vi "Process.vi"(8 "error in":errorcluster, 11 "Example Instrument UI":refnum<class "Instrument UI.Framework-Template.lvclass">) -> (0 "error out":errorcluster, 3 "Example Instrument UI out":refnum<class "Instrument UI.Framework-Template.lvclass">)   [LabVIEW 2019, in "Instrument UI.Framework-Template.lvclass"]
doc: "---------------------------------------------------------------\nJKI State Machine Objects™\nhttp://jki.net/state-machine-objects/\nCopyright (C) 2005-2015, JKI <info@jki.net>\nALL RIGHTS RESERVEDJKI State Machine Objects (SMO) 1.0.0.5\nJKI - JKI\nCopyright (c) 2016, JKI"
uses:
  Instrument UI.Framework-Template.lvclass
  C:/Program Files (x86)/National Instruments/LabVIEW 2019/vi.lib/JKI/JKI SMO/SMO/SMO.lvclass
  C:/Program Files (x86)/National Instruments/LabVIEW 2019/user.lib/LevyLab/Instrument Framework/SMOs/Instrument UI/Instrument UI.lvclass
  C:/Program Files (x86)/National Instruments/LabVIEW 2019/vi.lib/JKI/JKI SMO/SMO.UI/SMO.UI.lvclass
  Instrument.Framework-Template/Typedefs/Instrument.Framework-Template.getAll--Cluster.ctl
  Instrument.Framework-Template/Instrument.Framework-Template.lvclass
  C:/Program Files (x86)/National Instruments/LabVIEW 2019/user.lib/LevyLab/Instrument Framework/SMOs/Instrument/Instrument.lvclass
  Instrument UI.Framework-Template.UI--Cluster.ctl
  Instrument.Framework-Template/Typedefs/Instrument.Framework-Template.Configuration--Cluster.ctl
  <userlib>/LevyLab/Instrument Framework/SMOs/Configuration/Configuration.lvclass
  <userlib>/LevyLab/Instrument Framework/SMOs/Instrument UI/Instrument UI.lvclass/Instrument UI.ctl
  <vilib>/JKI/JKI SMO/SMO/SMO.lvclass/SMO.ctl
  <userlib>/LevyLab/Instrument Framework/SMOs/Configuration/Configuration.lvclass/Configuration.ctl
  <userlib>/LevyLab/Instrument Framework/SMOs/Instrument/Instrument.lvclass/Instrument.ctl
  <userlib>/LevyLab/Instrument Framework/SMOs/Instrument/Typedefs/Client Type--Enum.ctl
  614f1787-3484-4d72-b522-1f8c221dac07.vi
  064e3a37-d4cf-416d-9c97-81a00de9d50c.vi
  <vilib>/JKI/JKI SMO/SMO/Private/ReftoDVR--SMO.vi
  614f1787-3484-4d72-b522-1f8c221dac07.vi/6126265b-52a9-4036-b9ab-d7def26448fd.vi
  064e3a37-d4cf-416d-9c97-81a00de9d50c.vi/2934c5b6-9d9a-4612-aef0-474eff5135e3.vi
  614f1787-3484-4d72-b522-1f8c221dac07.vi/6126265b-52a9-4036-b9ab-d7def26448fd.vi/3777206e-62d3-4194-bbb6-d708f28c6636.vi
  <userlib>/LevyLab/Instrument Framework/SMOs/Instrument/API/Send and Receive.vi
  614f1787-3484-4d72-b522-1f8c221dac07.vi/6126265b-52a9-4036-b9ab-d7def26448fd.vi/c2acc09a-a3b2-411f-96f0-93bdcc04d904.vi
  <userlib>/LevyLab/Instrument Framework/SMOs/Instrument/Private/Get Client Type.vi
  064e3a37-d4cf-416d-9c97-81a00de9d50c.vi/2934c5b6-9d9a-4612-aef0-474eff5135e3.vi/d31bd197-f2cf-45ec-b348-66ecc1fb7fa3.vi
  064e3a37-d4cf-416d-9c97-81a00de9d50c.vi/2934c5b6-9d9a-4612-aef0-474eff5135e3.vi/bcf0d896-5092-4459-a902-822cb84f3d2f.vi
  614f1787-3484-4d72-b522-1f8c221dac07.vi/6126265b-52a9-4036-b9ab-d7def26448fd.vi/3777206e-62d3-4194-bbb6-d708f28c6636.vi/a171245e-ace2-4a31-ad0e-c1ba96aac09f.vi
  614f1787-3484-4d72-b522-1f8c221dac07.vi/6126265b-52a9-4036-b9ab-d7def26448fd.vi/3777206e-62d3-4194-bbb6-d708f28c6636.vi/314606e5-fab2-4c4b-855f-38e561406072.vi
  614f1787-3484-4d72-b522-1f8c221dac07.vi/6126265b-52a9-4036-b9ab-d7def26448fd.vi/c2acc09a-a3b2-411f-96f0-93bdcc04d904.vi/068c89fb-261c-4114-b3e0-8879b2039521.vi
  614f1787-3484-4d72-b522-1f8c221dac07.vi/6126265b-52a9-4036-b9ab-d7def26448fd.vi/c2acc09a-a3b2-411f-96f0-93bdcc04d904.vi/70e8e4d8-081c-4447-abab-7ffc08a24431.vi
  064e3a37-d4cf-416d-9c97-81a00de9d50c.vi/2934c5b6-9d9a-4612-aef0-474eff5135e3.vi/d31bd197-f2cf-45ec-b348-66ecc1fb7fa3.vi/16df6886-ccac-4f12-823d-852507d7b6d3.vi
  064e3a37-d4cf-416d-9c97-81a00de9d50c.vi/2934c5b6-9d9a-4612-aef0-474eff5135e3.vi/d31bd197-f2cf-45ec-b348-66ecc1fb7fa3.vi/d363edf0-f48d-4095-b52d-a98fc5c23e31.vi
  064e3a37-d4cf-416d-9c97-81a00de9d50c.vi/2934c5b6-9d9a-4612-aef0-474eff5135e3.vi/bcf0d896-5092-4459-a902-822cb84f3d2f.vi/3efd9854-12da-426d-b303-5f5dfdd99cd3.vi
  064e3a37-d4cf-416d-9c97-81a00de9d50c.vi/2934c5b6-9d9a-4612-aef0-474eff5135e3.vi/bcf0d896-5092-4459-a902-822cb84f3d2f.vi/021688bb-175a-4f04-92c2-7b75fc3f16e3.vi
  614f1787-3484-4d72-b522-1f8c221dac07.vi/6126265b-52a9-4036-b9ab-d7def26448fd.vi/c2acc09a-a3b2-411f-96f0-93bdcc04d904.vi/068c89fb-261c-4114-b3e0-8879b2039521.vi/f4340ad4-3f7d-43fc-a5b8-8cfecf0320e0.vi
  614f1787-3484-4d72-b522-1f8c221dac07.vi/6126265b-52a9-4036-b9ab-d7def26448fd.vi/c2acc09a-a3b2-411f-96f0-93bdcc04d904.vi/068c89fb-261c-4114-b3e0-8879b2039521.vi/09137493-ac28-451c-9813-f227a1b20a03.vi
  064e3a37-d4cf-416d-9c97-81a00de9d50c.vi/2934c5b6-9d9a-4612-aef0-474eff5135e3.vi/bcf0d896-5092-4459-a902-822cb84f3d2f.vi/3efd9854-12da-426d-b303-5f5dfdd99cd3.vi/ec8d0cc2-9f9f-4698-9277-550a01addf9f.vi
  064e3a37-d4cf-416d-9c97-81a00de9d50c.vi/2934c5b6-9d9a-4612-aef0-474eff5135e3.vi/bcf0d896-5092-4459-a902-822cb84f3d2f.vi/3efd9854-12da-426d-b303-5f5dfdd99cd3.vi/599ad89e-f603-4806-a637-659fe558540e.vi
  <userlib>/LevyLab/Instrument Framework/SMOs/Instrument/Private/Get RC Connection Status.vi
  <userlib>/LevyLab/Instrument Framework/SMOs/Instrument/API/Enum to String.vi
  <userlib>/LevyLab/Instrument Framework/SMOs/RemoteControl/API/Send and Receive.vi
  <vilib>/Utility/Data Type/Get Type Information.vi
  <vilib>/JDP Science/JSONtext/JSON text to Variant.vi
  <vilib>/JDP Science/JSONtext/Variant to JSON Text.vi
  <vilib>/National Instruments/GUID Generator/Guid Generator.vi
  <userlib>/LevyLab/Instrument Framework/SMOs/Instrument/Private/Instrument.MessageFromProcess.EventStructure.vi
  <userlib>/LevyLab/Instrument Framework/SMOs/Instrument/Instrument.lvclass
  <vilib>/JDP Science/JSONtext/LVClass Serializer/JSONtext LVClass Serializer.lvclass
  <userlib>/LevyLab/Instrument Framework/SMOs/Instrument UI/Instrument UI.lvclass
  <vilib>/JKI/JKI SMO/SMO/SMO.lvclass
  <vilib>/JKI/JKI SMO/SMO.UI/SMO.UI.lvclass
panel:
  in  "Parameter 2":string
  out "Numeric":u32
  in  "Set Parameter":bool
  in  "Parameter":dbl
  in  "STOP":bool
  out "SMO string":string
  out "SMO Boolean":bool
  out "Logger SMO":dbl
  out "Levy 1":dbl
  # "#todo\nmake UI here. maybe include a nice picture of the hardware?"
  # "#todo\nadd buttons to do stuff (e.g., change a setting)\nButtons should trigger an event"
  # "#todo\nresize this box if you want your UI to be different size"
  # "SMO UI Template"
  # "For instructions on how to use the JKI State Machine Objects, examples and video tutorials, visit:\nhttp://jki.net/state-machine-objects/\n\nJKI State Machine Objects™\nhttp://jki.net/state-machine-objects/\nCopyright (C) 2005-2015, JKI <info@jki.net>\nALL RIGHTS RESERVED"
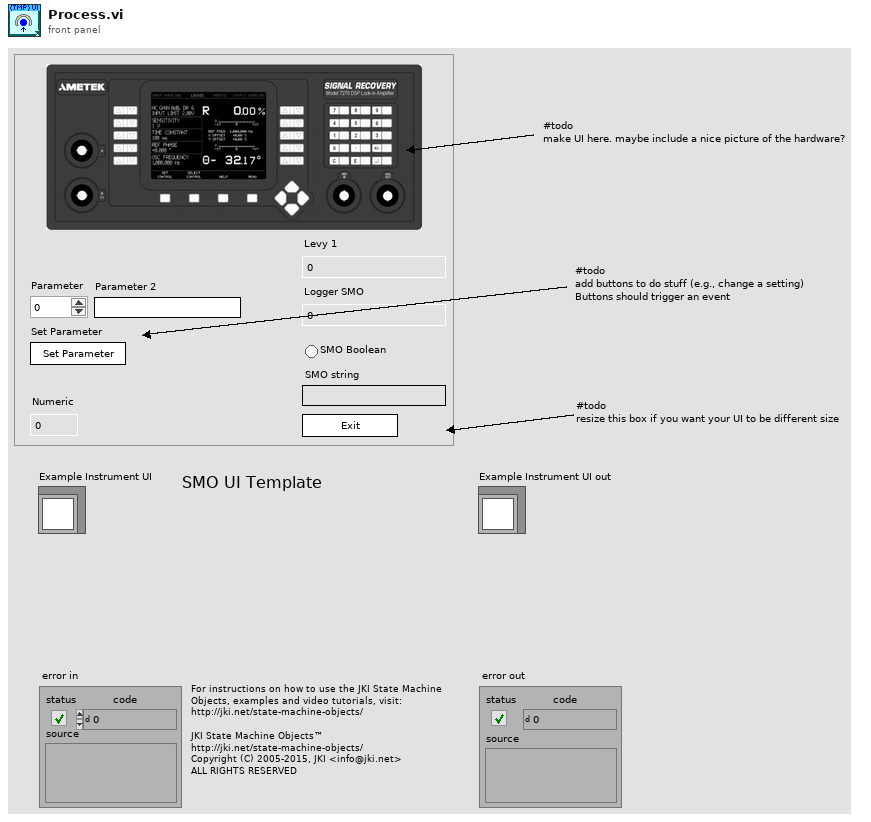
[diagram p1: front panel]
types:
  T1 = enum32{"invalid app kind", "Development System", "Run Time System", "Student Edition", "Embedded LabVIEW", "Evaluation", "Custom"}
  T2 = enum32{"Invalid", "Standard", "Closed", "Hidden", "Minimized", "Maximized"}
  T3 = typedef "Instrument.lvclass/Client Type--Enum.ctl" = enum16{"Remote", "Local"}
  T4 = typedef "Instrument.Framework-Template.lvclass/Instrument.Framework-Template.Configuration--Cluster.ctl" = cluster{"Example Setting 1":dbl, "Example Setting 2":dbl, "Example Setting 3":string}
  T5 = typedef "Instrument.Framework-Template.lvclass/Instrument.Framework-Template.getAll--Cluster.ctl" = cluster{"Levy 1":dbl, "Logger SMO":dbl, "SMO Boolean":bool, "SMO String":string}
  T6 = typedef "Instrument UI.Framework-Template.lvclass/Instrument UI.Framework-Template.UI--Cluster.ctl" = cluster{"Parameter":dbl, "Parameter 2":string}
  T7 = cluster{"Core":cluster{"Current VI Reference":refnum<vi>, "Close Panel on Exit?":bool, "Last Error":cluster{"error":errorcluster, "previous state":string, "remaining states":string}, "Shutdown?":bool}, "Instrument UI":refnum<class "Instrument UI.Framework-Template.lvclass">, "Instrument":refnum<class "Instrument.Framework-Template.lvclass">, "Configuration":refnum<class "Configuration.lvclass">, "Config Cluster":T4, "getAll":T5, "UI Cluster":T6}
  T8 = cluster{"Current VI Reference":refnum<vi>, "Close Panel on Exit?":bool, "Last Error":cluster{"error":errorcluster, "previous state":string, "remaining states":string}, "Shutdown?":bool}
  T9 = typedef "SMO.lvclass/Protected Events.ctl" = cluster{"StopProcesses":refnum<user-event>, "AbortProcesses":refnum<user-event>, "Config Changed":refnum<user-event>, "Dependency":refnum<user-event>}
  T10 = typedef "Instrument.lvclass/PublicEvents--Cluster.ctl" = cluster{"MessageFromProcess":refnum<user-event>}
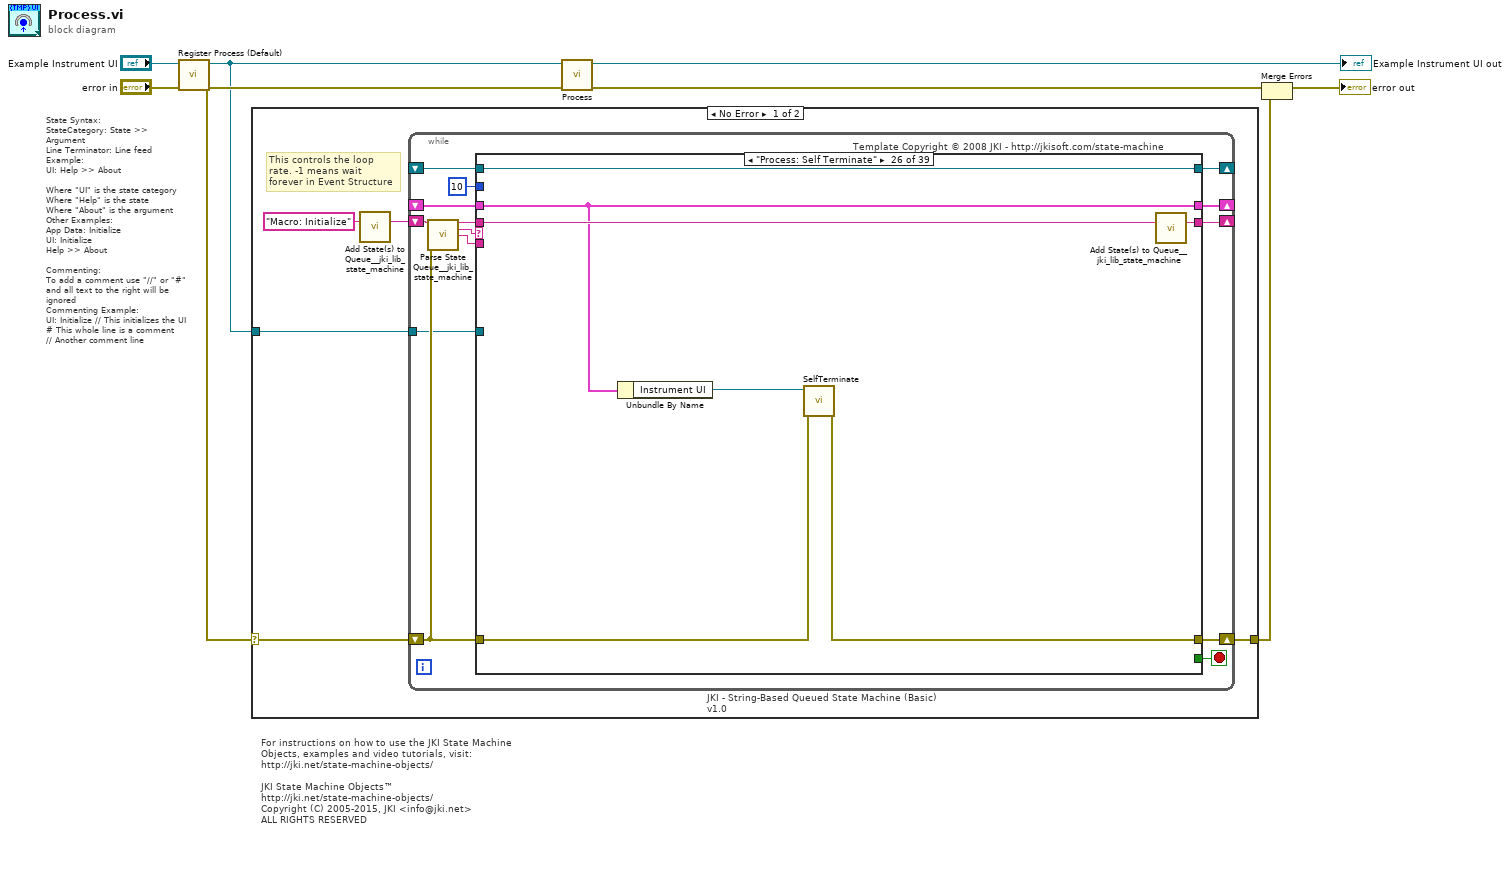
[diagram p0: block diagram]
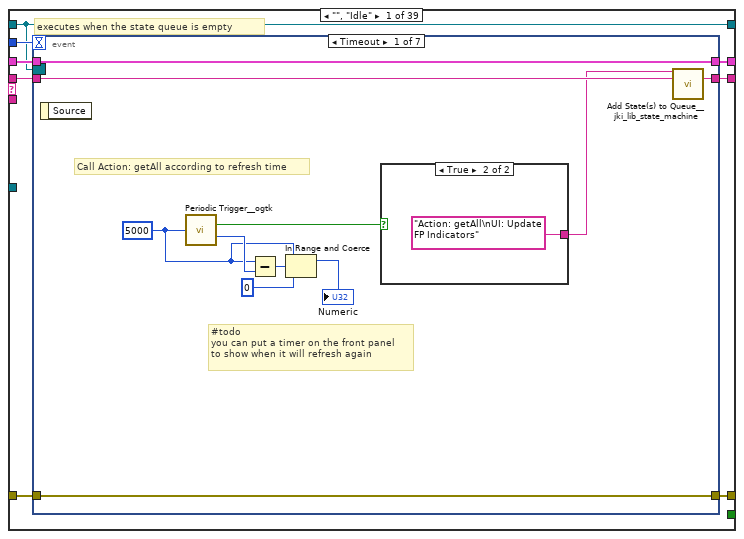
[diagram p2: hidden frame]
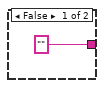
[diagram p3: hidden frame]
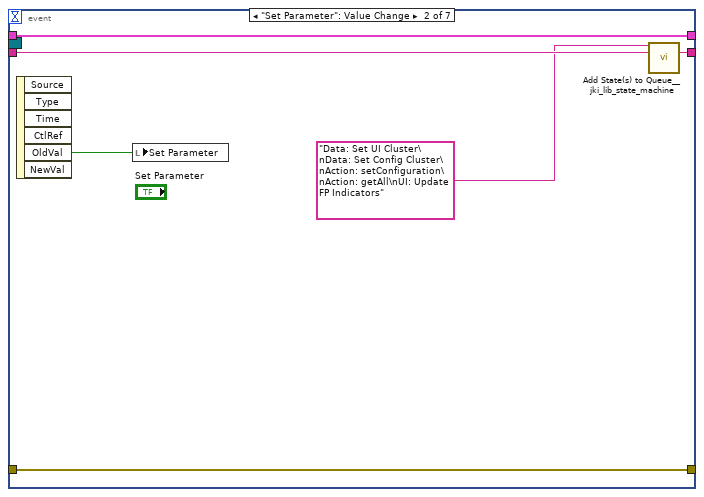
[diagram p4: hidden frame]
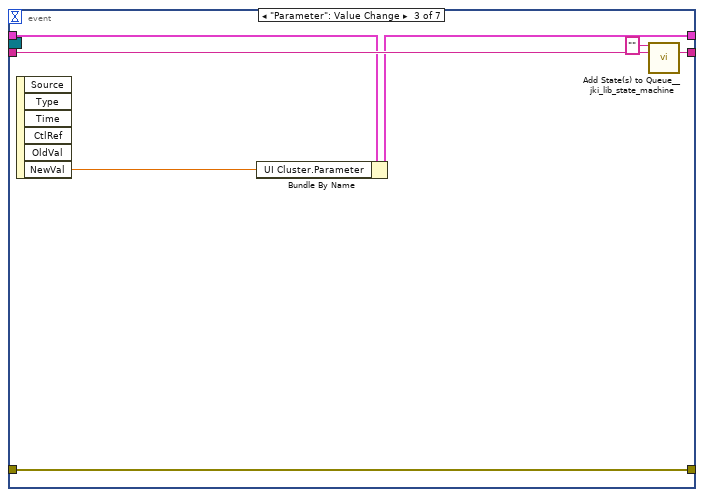
[diagram p5: hidden frame]
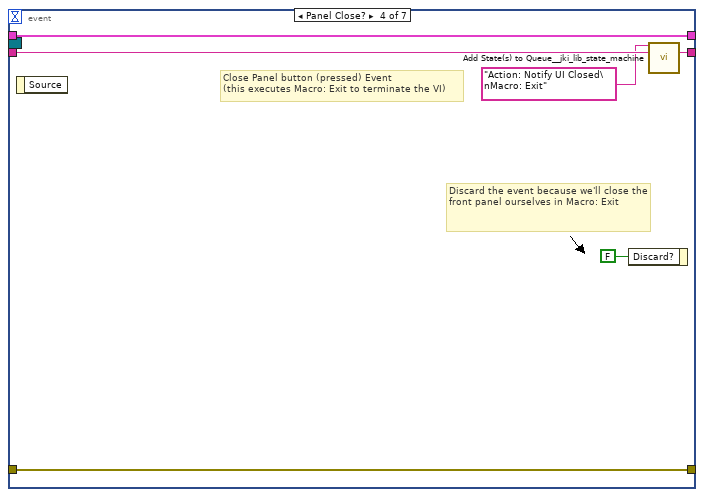
[diagram p6: hidden frame]
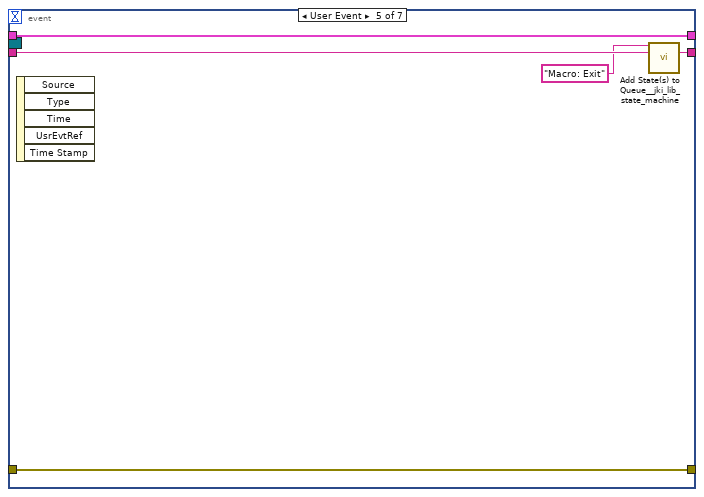
[diagram p7: hidden frame]
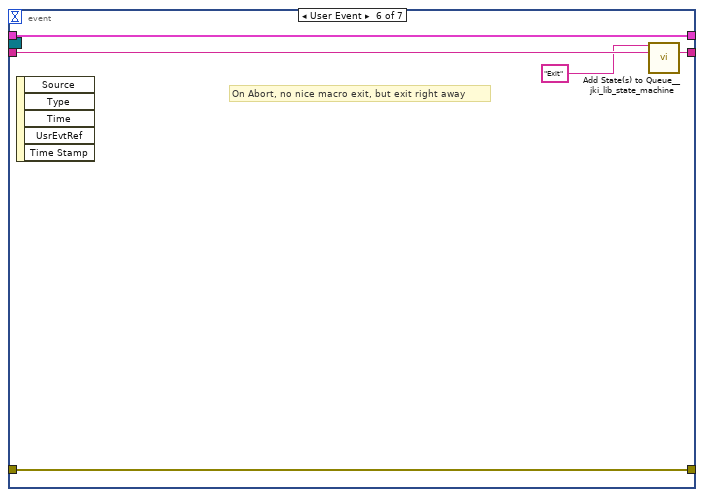
[diagram p8: hidden frame]
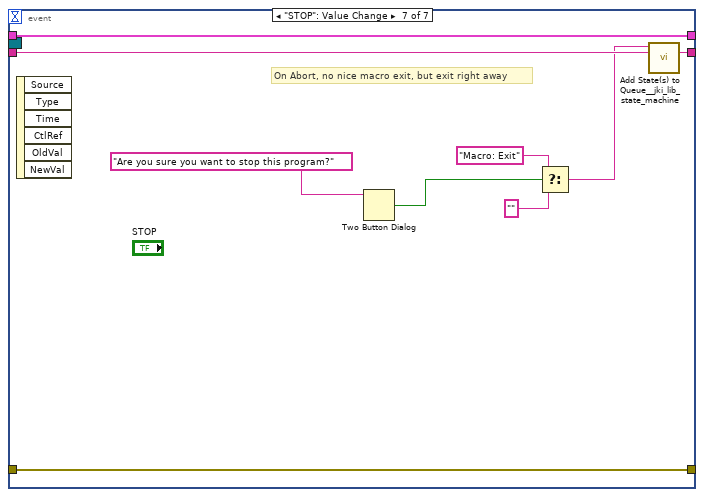
[diagram p9: hidden frame]
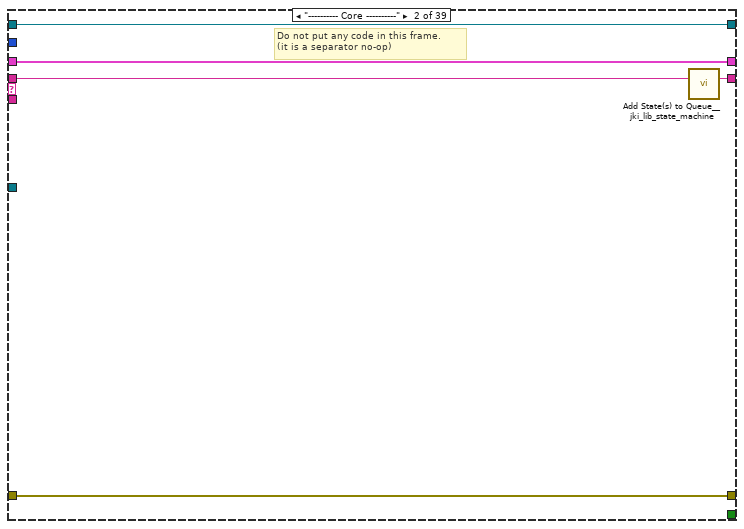
[diagram p10: hidden frame]
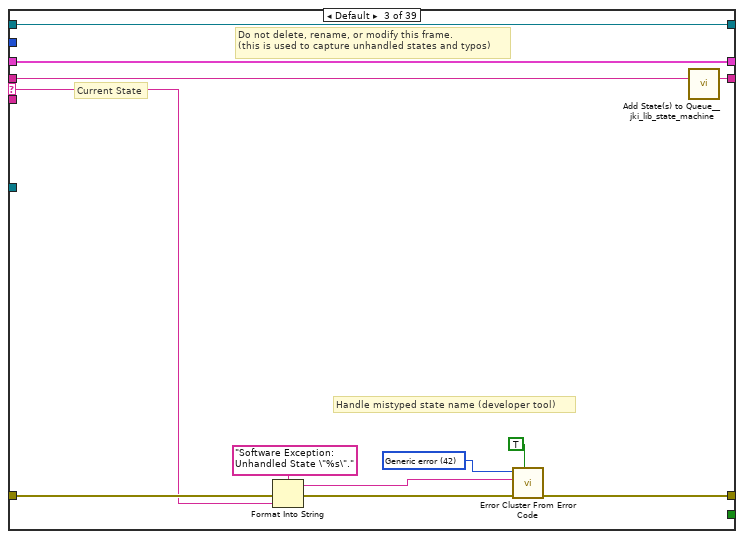
[diagram p11: hidden frame]
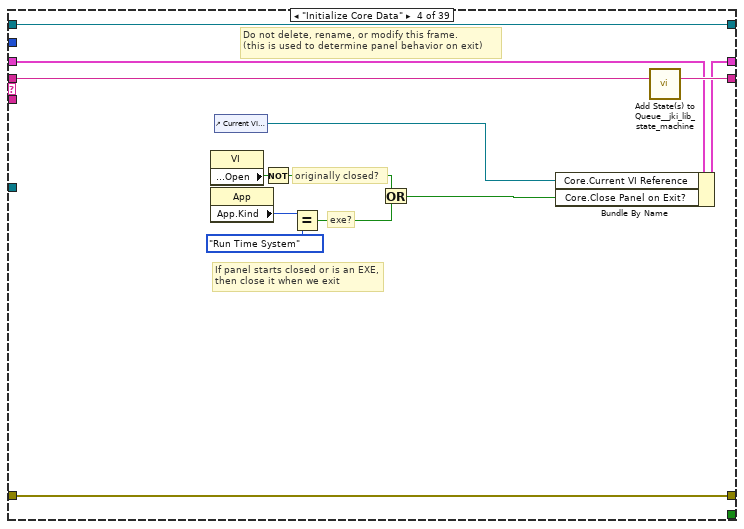
[diagram p12: hidden frame]
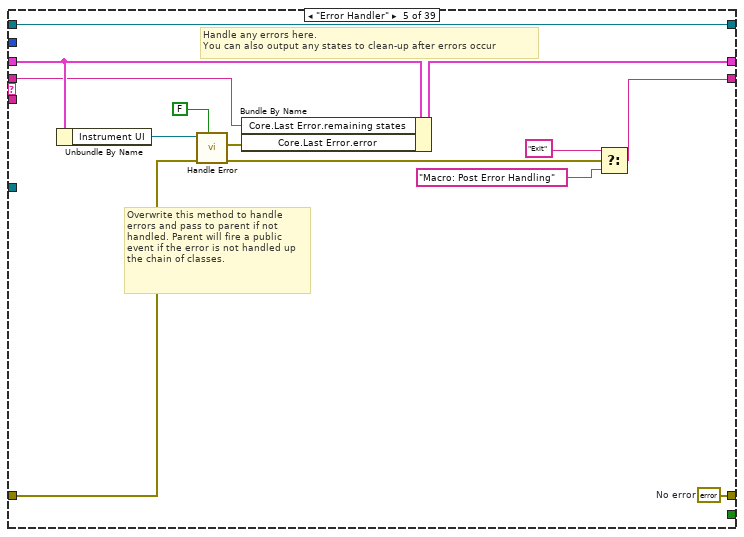
[diagram p13: hidden frame]
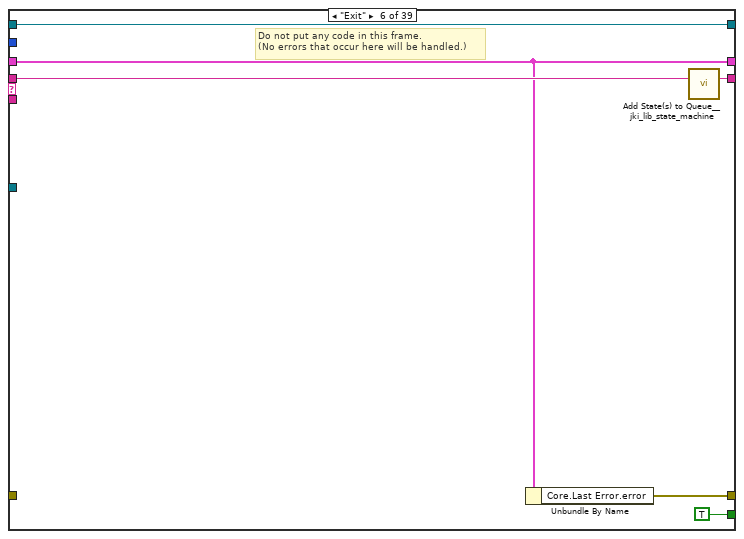
[diagram p14: hidden frame]
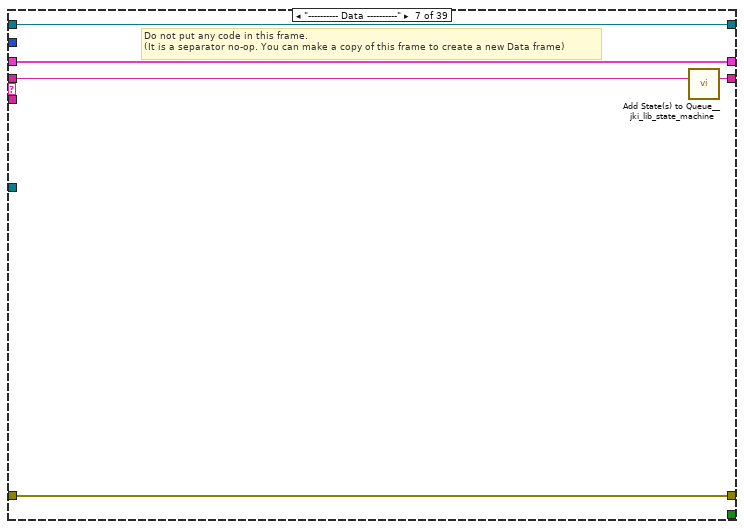
[diagram p15: hidden frame]
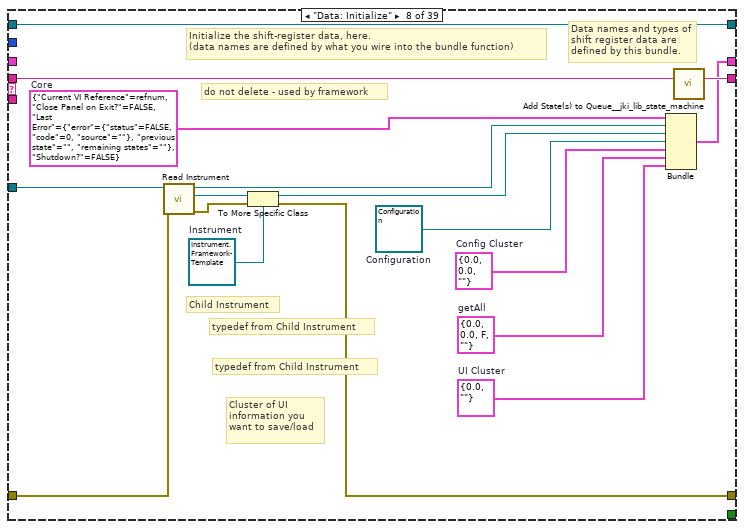
[diagram p16: hidden frame]
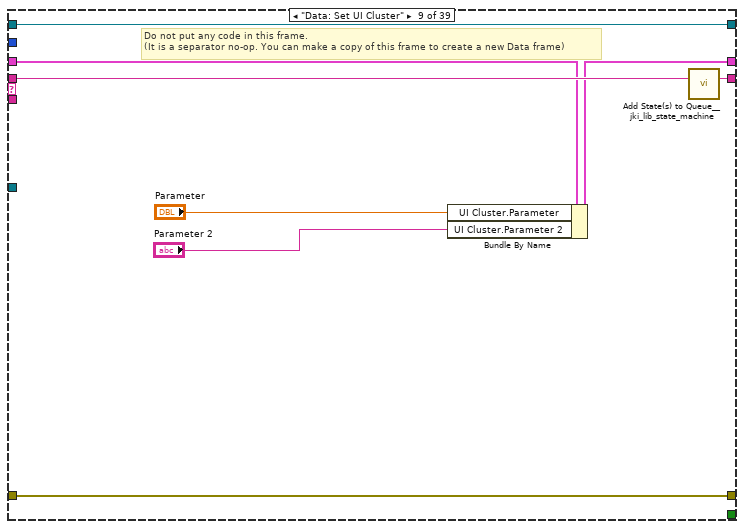
[diagram p17: hidden frame]
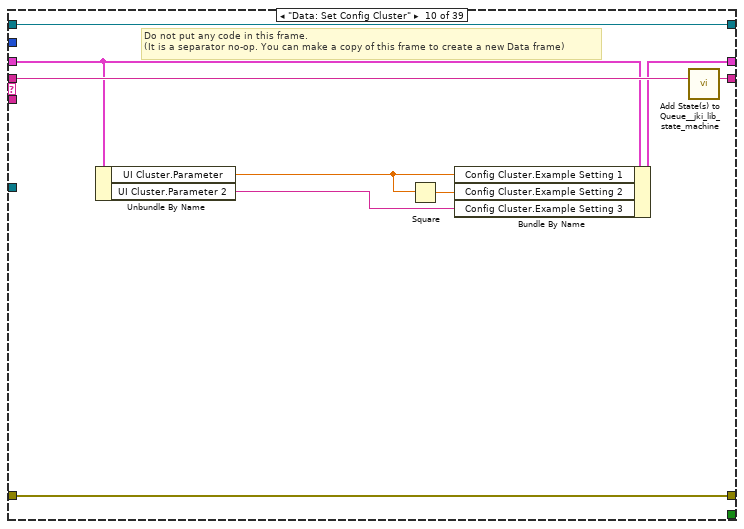
[diagram p18: hidden frame]
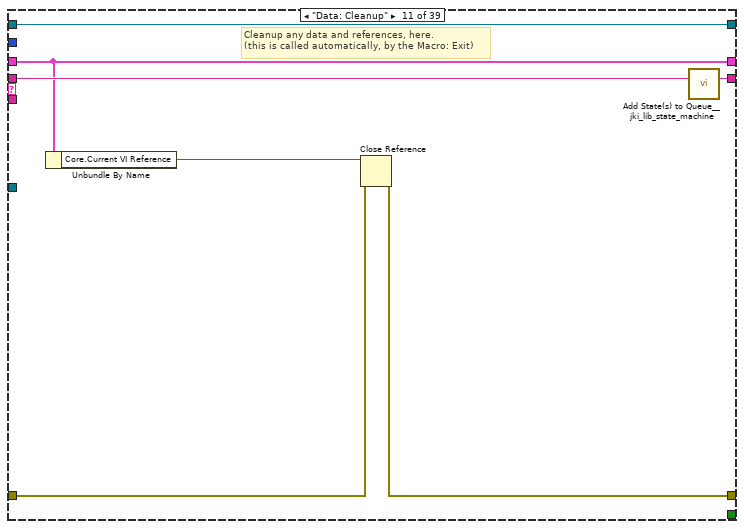
[diagram p19: hidden frame]
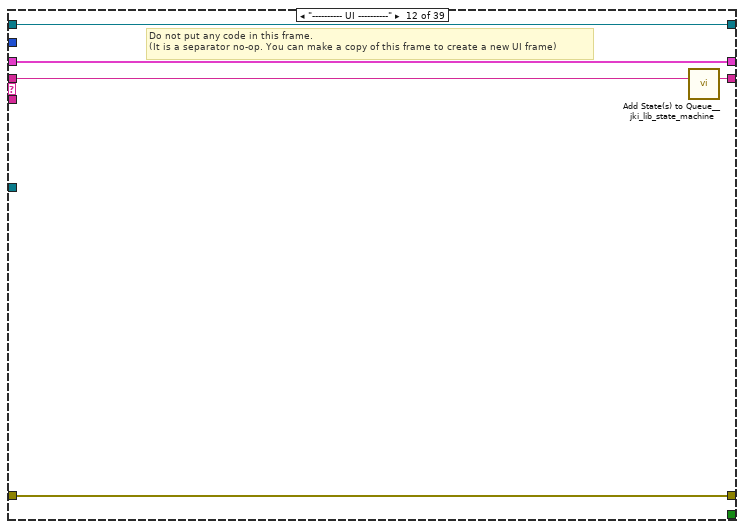
[diagram p20: hidden frame]
diagram:
  # "State Syntax:\nStateCategory: State >> Argument\nLine Terminator: Line feed\nExample:\nUI: Help >> About\n\nWhere \"UI\" is the state category\nWhere \"Help\" is the state\nWhere \"About\" is the argument\nOther Examples:\nApp Data: Initialize\nUI: Initialize\nHelp >> About\n\nCommenting:\nTo add a comment use \"//\" or \"#\" and all text to the right will be ignored\nCommenting Example:\nUI: Initialize // This initializes the UI\n# This whole line is a comment\n// Another comment line"
  # "For instructions on how to use the JKI State Machine Objects, examples and video tutorials, visit:\nhttp://jki.net/state-machine-objects/\n\nJKI State Machine Objects™\nhttp://jki.net/state-machine-objects/\nCopyright (C) 2005-2015, JKI <info@jki.net>\nALL RIGHTS RESERVED"
  n1 = call <vilib>:"Register Process (Default).vi"("error in (no error)"="error in", "SMO"="Example Instrument UI") -> ("error out"=w5:errorcluster, "SelfRef"=w4:refnum<class "Instrument UI.Framework-Template.lvclass">)  [unwired: 8 in]
  n2 = case shown="No Error" w5 {
    selector: w5 -> [w10 w465]
    tunnel: w4 -> [w11 _]
    tunnel: [w9 w465] -> w1
    frame No Error {
      # "This controls the loop rate. -1 means wait forever in Event Structure"
      n3 = call <vilib>:"Add State(s) to Queue__jki_lib_state_machine.vi"("State(s) in (\"\")"="Macro: Initialize") -> ("States Out"=w13:string)  [unwired: 14 in]
      n4 = while "JKI - String-Based Queued State Machine (Basic) v1.0" {
        shift-right: [w20] -> _
        shift-left: _ -> [w19]
        shift-right: [w23] -> w9
        shift-left: w10 -> [w17]
        shift-right: [w22] -> _
        shift-left: w13 -> [w24]
        tunnel: w11 -> [w16]
        shift-right: [w15] -> _
        shift-left: _ -> [w14]
        stop <- w21 stop-if-true
        # "Template Copyright © 2008 JKI - http://jkisoft.com/state-machine"
        n5 = call <vilib>:"Parse State Queue__jki_lib_state_machine.vi"("State Queue"=w24, "Error In (no error)"=w17) -> ("Remaining States"=w26:string, "Current State"=w27:string, "Arguments"=w25:string)  [unwired: 11 in]
        n6 = case shown="\"Process: Self Terminate\"" w27 {
          selector: w27 -> [_ _ w93 _ _ _ _ _ _ _ _ _ _ _ _ _ _ _ _ _ _ _ _ _ _ _ _ _ _ _ _ _ _ _ _ _ _ _ _]
          tunnel: w26 -> [w35 w91 w97 w116 w120 w135 w140 w157 w165 w174 w181 w186 w193 w200 w210 w217 w233 w265 w274 w286 w296 w302 w317 w322 w333 w340 w345 w358 w364 w369 w384 w392 w404 w411 w418 w430 w443 w453 w464]
          tunnel: w25 -> [_ _ _ _ _ _ _ _ _ _ _ _ _ _ _ w211 w227 _ _ _ _ _ _ _ _ _ _ _ _ _ _ _ _ _ _ _ _ _ _]
          tunnel: w19 -> [w33 w88 w95 w107 w123 w131 w137 _ w161 w170 w175 w183 w191 w196 w201 w215 w229 w262 w270 w276 w293 w299 w304 w319 w330 w335 w342 w356 w362 w366 w377 w389 w395 w407 w412 w422 w437 w445 w456]
          tunnel: [w32 w89 w99 w113 w125 w130 w138 w144 w163 w172 w177 w184 w188 w198 w202 w212 w230 w263 w272 w284 w294 w300 w315 w320 w324 w336 w343 w351 w359 w367 w370 w387 w396 w408 w413 w427 w440 w450 w461] -> w23
          tunnel: w17 -> [w31 w89 w98 w113 w119 _ w138 w141 w163 w172 w178 w184 w189 w198 w202 w213 w231 w263 w272 w284 w294 w300 w315 w320 w325 w337 w343 w353 w360 w367 w379 w385 w397 w408 w414 w423 w432 w446 w457]
          tunnel: [w34 w90 w96 w115 w117 w134 w139 w156 w164 w173 w180 w185 w192 w199 w209 w216 w232 w264 w273 w285 w295 w301 w316 w321 w332 w339 w344 w357 w363 w368 w383 w391 w403 w410 w417 w429 w442 w452 w463] -> w22
          tunnel: [_ _ _ _ _ TRUE _ _ _ _ _ _ _ _ _ _ _ _ _ _ _ _ _ _ _ _ _ _ _ _ _ _ _ _ _ _ _ _ _] -> w21
          tunnel: [w30 w88 w95 w114 w122 w131 w137 w155 w160 w169 w175 w183 w191 w196 w201 w215 w229 w262 w270 w277 w293 w299 w304 w319 w330 w335 w342 w356 w362 w366 w381 w389 w393 w406 w412 w424 w438 w447 w458] -> w20
          tunnel: 10 ("Timeout") -> [w29 _ _ _ _ _ _ _ _ _ _ _ _ _ _ _ _ _ _ _ _ _ _ _ _ _ _ _ _ _ _ _ _ _ _ _ _ _ _]
          tunnel: w16 -> [_ _ _ _ _ _ _ w142 _ _ _ _ _ _ _ _ _ _ _ _ _ _ _ _ _ _ _ _ _ _ _ _ _ _ _ _ _ _ _]
          tunnel: [w28 w87 w92 w104 w129 w132 w136 w154 w162 w171 w176 w182 w190 w197 w208 w214 w226 w261 w271 w283 w292 w298 w309 w318 w331 w338 w341 w355 w361 w365 w382 w390 w402 w409 w416 w428 w441 w451 w462] -> w15
          tunnel: w14 -> [w28 w87 w92 w104 w129 w132 w136 w154 w162 w171 w176 w182 w190 w197 w208 w214 w226 w261 w271 w283 w292 w298 w309 w318 w331 w338 w341 _ w361 w365 w382 w390 w402 w409 w416 w428 w441 w451 w462]
          frame "", "Idle" {
            # "executes when the state queue is empty"
            n7 = event shown="[0] Timeout" {
              selector: w28 -> [_ _ _ _ _ _ _]
              dyn-events: _ -> [_ _ _ _ _ _ _]
              timeout: w29 -> [_ _ _ _ _ _ _]
              tunnel: w35 -> [w46 w54 w61 w67 w72 w77 w86]
              tunnel: [w45 w53 w60 w66 w71 w76 w85] -> w34
              tunnel: w33 -> [w43 w51 w57 w63 w69 w74 w83]
              tunnel: [w44 w52 w59 w62 w70 w75 w84] -> w32
              tunnel: w31 -> [w44 w52 w59 w62 w70 w75 w84]
              tunnel: [w43 w51 w56 w63 w69 w74 w83] -> w30
              event Timeout {
                w37 = u32 5000 ("time (ms)")
                # "#todo\nyou can put a timer on the front panel\nto show when it will refresh again"
                # "Call Action: getAll according to refresh time"
                n8 = event-data() -> ()  [unwired: 1 in, 1 out]
                n9 = call <userlib>:"Periodic Trigger__ogtk.vi"("time (ms)"=w37) -> ("Triggered"=w41:bool, "timer value"=w40:u32)  [unwired: 12 in, 1 out]
                n10 = Subtract(x=w37, y=w40) -> (x-y=w39:u32)
                n11 = In Range and Coerce(upper limit=w37, x=w39, lower limit=u32 0) -> (coerced(x)=→"Numeric":u32)  [unwired: 1 out]
                n12 = case shown="True" w41 {
                  tunnel: ["" ("State(s) in Front (\"\")") "Action: getAll\nUI: Update FP Indicators" ("State(s) in Front (\"\")")] -> w42
                  frame False {
                  }
                  frame True {
                  }
                }
                n13 = call <vilib>:"Add State(s) to Queue__jki_lib_state_machine.vi"("State(s) in Front (\"\")"=w42, "State(s) in (\"\")"=w46) -> ("States Out"=w45:string)  [unwired: 13 in]
              }
              event "Set Parameter": Value Change {
                n14 = event-data() -> ("OldVal"=w50:bool)  [unwired: 1 in, 5 out]
                n15 = local write "Set Parameter"(w50) -> ()
                n16 = call <vilib>:"Add State(s) to Queue__jki_lib_state_machine.vi"("State(s) in Front (\"\")"="Data: Set UI Cluster\nData: Set Config Cluster\nAction: setConfiguration\nAction: getAll\nUI: Update FP Indicators" ("State(s) in Front (\"\")"), "State(s) in (\"\")"=w54) -> ("States Out"=w53:string)  [unwired: 13 in]
              }
              event "Parameter": Value Change {
                n17 = event-data() -> ("NewVal"=w58:dbl)  [unwired: 1 in, 5 out]
                n18 = Bundle By Name(cluster=w57, "UI Cluster.Parameter"=w58) -> (w56:T7)
                n19 = call <vilib>:"Add State(s) to Queue__jki_lib_state_machine.vi"("State(s) in Front (\"\")"="" ("State(s) in Front (\"\")"), "State(s) in (\"\")"=w61) -> ("States Out"=w60:string)  [unwired: 13 in]
              }
              event Panel Close? {
                # "Discard the event because we'll close the front panel ourselves in Macro: Exit"
                # "Close Panel button (pressed) Event\n(this executes Macro: Exit to terminate the VI)"
                n20 = event-data() -> ()  [unwired: 1 in, 1 out]
                n21 = event-data("Discard?"=FALSE) -> ()  [unwired: 1 in, 1 out]
                n22 = call <vilib>:"Add State(s) to Queue__jki_lib_state_machine.vi"("State(s) in Front (\"\")"="Action: Notify UI Closed\nMacro: Exit", "State(s) in (\"\")"=w67) -> ("States Out"=w66:string)  [unwired: 13 in]
              }
              event User Event {
                n23 = event-data() -> ()  [unwired: 1 in, 5 out]
                n24 = call <vilib>:"Add State(s) to Queue__jki_lib_state_machine.vi"("State(s) in Front (\"\")"="Macro: Exit", "State(s) in (\"\")"=w72) -> ("States Out"=w71:string)  [unwired: 13 in]
              }
              event User Event {
                # "On Abort, no nice macro exit, but exit right away"
                n25 = event-data() -> ()  [unwired: 1 in, 5 out]
                n26 = call <vilib>:"Add State(s) to Queue__jki_lib_state_machine.vi"("State(s) in Front (\"\")"="Exit", "State(s) in (\"\")"=w77) -> ("States Out"=w76:string)  [unwired: 13 in]
              }
              event "STOP": Value Change {
                # "On Abort, no nice macro exit, but exit right away"
                n27 = event-data() -> ()  [unwired: 1 in, 6 out]
                n28 = Two Button Dialog(message="Are you sure you want to stop this program?") -> (T button?=w82:bool)  [unwired: 2 in]
                n29 = Select(t="Macro: Exit", s=w82, f="") -> (s? t:f=w78:string)
                n30 = call <vilib>:"Add State(s) to Queue__jki_lib_state_machine.vi"("State(s) in Front (\"\")"=w78, "State(s) in (\"\")"=w86) -> ("States Out"=w85:string)  [unwired: 13 in]
              }
            }
          }
          frame "---------- Core ----------" {
            # "Do not put any code in this frame.\n(it is a separator no-op)"
            n31 = call <vilib>:"Add State(s) to Queue__jki_lib_state_machine.vi"("State(s) in (\"\")"=w91) -> ("States Out"=w90:string)  [unwired: 14 in]
          }
          frame Default {
            w102 = 42 items=["No error", "Argument error", "Memory is full", "Out of zone", "End of file", "File already open", "Generic file I/O error", "File not found", "File permission error", "Disk is full", "Duplicate path", "Too many files open", "System feature not enabled", "Resource file not found", "Cannot add resource", "Resource not found", "Image not found", "Image memory error", "Pen does not exist", "Config type invalid", "Config token not found", "Config parse error", "Config memory error", "Bad external code format", "Bad external code offset", "External code not present", "Null window", "Destroy window error", "Null menu", "Print aborted", "Bad print record", "Print driver error", "Windows error during printing", "Memory error during printing", "Print dialog error", "Generic print error", "Invalid device refnum", "Device not found", "Device parameter error", "Device unit error", "Cannot open device", "Device call aborted", "Generic error", "Cancelled by user", "Object ID too low", "Object ID too high", "Object not in heap", "Unknown heap", "Unknown object (invalid DefProc)", "Unknown object (DefProc not in table)", "Message out of range", "Invalid (null) method", "Unknown message", "Manager call not supported", "Bad address", "Network operation in progress", "Network operation timed out", "Connection is busy", "Network attribute not supported", "Network error", "Address in use", "System out of memory", "Connection aborted", "Connection refused", "Not connected", "Already connected", "Connection closed", "Initialization error (interapplication manager)", "Bad occurrence", "Wait on unbound occurrence handler", "Occurrence queue overflow", "Datalog type conflict", "Unused", "Unrecognized type (interapplication manager)", "Memory corrupt", "Failed to make temporary DLL", "Old CIN version", "Drag socket not found", "Failed to load drop-object", "Failed to register OLE object", "Failed to release OLE object", "Format specifier type mismatch", "Unknown format specifier", "Too few format specifiers", "Too many format specifiers", "Scan failed", "Newer CIN version", "Error converting to variant", "Runtime menu error", "Password tampered", "Variant attribute not found", "Incompatible variant data type", "Event data is not available", "Event Store is not present", "Occurrence is not found", "Event Queue is not created", "Event info is not available", "Refnum passed is NULL", "Error retrieving Class GUID", "Error retrieving CoClass GUID", "Error retrieving TypeLib GUID.", "Bad built application magic bytes.", "Specific driver is different from the specific driver associated with the Logical Name.", "There is no session opened to the class driver.", "Max Error", "MAX - Error with config objects", "MAX - Error loading configuration", "MAX - Group not supported"]
            # "Current State"
            # "Do not delete, rename, or modify this frame.\n(this is used to capture unhandled states and typos)"
            # "Handle mistyped state name (developer tool)"
            n32 = Format Into String(format string="Software Exception: Unhandled State \"%s\"." ("message"), error in=w98, w93) -> (resulting string=w101:string, error out=w100:errorcluster)  [unwired: 1 in]
            n33 = call <vilib>:"Error Cluster From Error Code.vi"("show call chain? (False)"=TRUE, "error in (no error)"=w100, "error message (\"\")"=w101, "error code (0)"=w102) -> ("error out"=w99:errorcluster)  [unwired: 5 in]
            n34 = call <vilib>:"Add State(s) to Queue__jki_lib_state_machine.vi"("State(s) in (\"\")"=w97) -> ("States Out"=w96:string)  [unwired: 14 in]
          }
          frame "Initialize Core Data" {
            # "Do not delete, rename, or modify this frame.\n(this is used to determine panel behavior on exit)"
            # "originally closed?"
            # "exe?"
            # "If panel starts closed or is an EXE, then close it when we exit"
            n35 = property class="VI"() -> ("Front Panel.Open"=w112:bool)  [unwired: 2 in, 2 out]
            n36 = property class="App"() -> ("App.Kind"=w111:T1)  [unwired: 2 in, 2 out]
            n37 = control-ref of="Current VI Reference"() -> (w105:refnum<vi>)
            n38 = Not(x=w112) -> (.not. x?=w109:bool)
            n39 = Equal?(x=w111, y=T1."Run Time System" ("Application:Kind")) -> (x = y?=w108:bool)
            n40 = Or(x=w109, y=w108) -> (x .or. y?=w106:bool)
            n41 = Bundle By Name(cluster=w107, "Core.Current VI Reference"=w105, "Core.Close Panel on Exit?"=w106) -> (w114:T7)
            n42 = call <vilib>:"Add State(s) to Queue__jki_lib_state_machine.vi"("State(s) in (\"\")"=w116) -> ("States Out"=w115:string)  [unwired: 14 in]
          }
          frame "Error Handler" {
            w125 = errorcluster {"status"=FALSE, "code"=0, "source"=""}  # No error
            # "Overwrite this method to handle errors and pass to parent if not handled. Parent will fire a public event if the error is not handled up the chain of classes."
            # "Handle any errors here.\nYou can also output any states to clean-up after errors occur"
            n43 = Unbundle By Name(w123) -> ("Instrument UI"=w128:refnum<class "Instrument UI.Framework-Template.lvclass">)
            n44 = call-dynamic "Handle Error.vi"("Stop on Unhandled Error (T)"=FALSE, "error in"=w119, "SMO"=w128) -> ("handling error"=w126:errorcluster, "Unhandled error"=w124:errorcluster)  [unwired: 6 in, 1 out]
            n45 = Bundle By Name(cluster=w123, "Core.Last Error.remaining states"=w120, "Core.Last Error.error"=w124) -> (w122:T7)
            n46 = Select(t="Exit", s=w126, f="Macro: Post Error Handling") -> (s? t:f=w117:string)
          }
          frame "Exit" {
            # "Do not put any code in this frame.\n(No errors that occur here will be handled.)"
            n47 = Unbundle By Name(w131) -> ("Core.Last Error.error"=w130:errorcluster)
            n48 = call <vilib>:"Add State(s) to Queue__jki_lib_state_machine.vi"("State(s) in (\"\")"=w135) -> ("States Out"=w134:string)  [unwired: 14 in]
          }
          frame "---------- Data ----------" {
            # "Do not put any code in this frame.\n(It is a separator no-op. You can make a copy of this frame to create a new Data frame)"
            n49 = call <vilib>:"Add State(s) to Queue__jki_lib_state_machine.vi"("State(s) in (\"\")"=w140) -> ("States Out"=w139:string)  [unwired: 14 in]
          }
          frame "Data: Initialize" {
            w143 = refnum<class "Configuration.lvclass"> refnum  # Configuration
            w146 = T4 {"Example Setting 1"=0.0, "Example Setting 2"=0.0, "Example Setting 3"=""}  # Config Cluster
            w148 = T6 {"Parameter"=0.0, "Parameter 2"=""}  # UI Cluster
            w150 = refnum<class "Instrument.Framework-Template.lvclass"> refnum  # Instrument
            w152 = T5 {"Levy 1"=0.0, "Logger SMO"=0.0, "SMO Boolean"=FALSE, "SMO String"=""}  # getAll
            w153 = T8 {"Current VI Reference"=refnum, "Close Panel on Exit?"=FALSE, "Last Error"={"error"={"status"=FALSE, "code"=0, "source"=""}, "previous state"="", "remaining states"=""}, "Shutdown?"=FALSE}  # Core
            # "typedef from Child Instrument"
            # "Cluster of UI\ninformation you\nwant to save/load"
            # "Child Instrument"
            # "typedef from Child Instrument"
            # "do not delete - used by framework"
            # "Data names and types of shift register data are defined by this bundle."
            # "Initialize the shift-register data, here.\n(data names are defined by what you wire into the bundle function)"
            n50 = call <userlib>:"Read Instrument.vi"("error in (no error)"=w141, "Instrument UI in"=w142) -> ("error out"=w147:errorcluster, "Instrument"=w149:refnum<class "Instrument.lvclass">, "Instrument UI"=w151:refnum<class "Instrument UI.Framework-Template.lvclass">)  [unwired: 7 in]
            n51 = To More Specific Class(target class=w150, reference=w149, error in=w147) -> (specific class reference=w145:refnum<class "Instrument.Framework-Template.lvclass">, error out=w144:errorcluster)
            n52 = Bundle("Core"=w153, "Instrument UI"=w151, "Instrument"=w145, "Configuration"=w143, "Config Cluster"=w146, "getAll"=w152, "UI Cluster"=w148) -> (w155:T7)  [unwired: 1 in]
            n53 = call <vilib>:"Add State(s) to Queue__jki_lib_state_machine.vi"("State(s) in (\"\")"=w157) -> ("States Out"=w156:string)  [unwired: 14 in]
          }
          frame "Data: Set UI Cluster" {
            # "Do not put any code in this frame.\n(It is a separator no-op. You can make a copy of this frame to create a new Data frame)"
            n54 = Bundle By Name(cluster=w161, "UI Cluster.Parameter"="Parameter", "UI Cluster.Parameter 2"="Parameter 2") -> (w160:T7)
            n55 = call <vilib>:"Add State(s) to Queue__jki_lib_state_machine.vi"("State(s) in (\"\")"=w165) -> ("States Out"=w164:string)  [unwired: 14 in]
          }
          frame "Data: Set Config Cluster" {
            # "Do not put any code in this frame.\n(It is a separator no-op. You can make a copy of this frame to create a new Data frame)"
            n56 = Unbundle By Name(w170) -> ("UI Cluster.Parameter"=w167:dbl, "UI Cluster.Parameter 2"=w168:string)
            n57 = Square(x=w167) -> (x^2=w166:dbl)
            n58 = Bundle By Name(cluster=w170, "Config Cluster.Example Setting 1"=w167, "Config Cluster.Example Setting 2"=w166, "Config Cluster.Example Setting 3"=w168) -> (w169:T7)
            n59 = call <vilib>:"Add State(s) to Queue__jki_lib_state_machine.vi"("State(s) in (\"\")"=w174) -> ("States Out"=w173:string)  [unwired: 14 in]
          }
          frame "Data: Cleanup" {
            # "Cleanup any data and references, here.\n(this is called automatically, by the Macro: Exit)"
            n60 = Unbundle By Name(w175) -> ("Core.Current VI Reference"=w179:refnum<vi>)
            n61 = Close Reference(reference=w179, error in (no error)=w178) -> (error out=w177:errorcluster)
            n62 = call <vilib>:"Add State(s) to Queue__jki_lib_state_machine.vi"("State(s) in (\"\")"=w181) -> ("States Out"=w180:string)  [unwired: 14 in]
          }
          frame "---------- UI ----------" {
            # "Do not put any code in this frame.\n(It is a separator no-op. You can make a copy of this frame to create a new UI frame)"
            n63 = call <vilib>:"Add State(s) to Queue__jki_lib_state_machine.vi"("State(s) in (\"\")"=w186) -> ("States Out"=w185:string)  [unwired: 14 in]
          }
          frame "UI: Initialize" {
            # "size window to decoration box on front panel"
            # "Initialize the User Interface, here.\n(this is called automatically, by the Macro: Init)"
            n64 = invoke on="STOP" class="Bool (strict)" method="Reinit To Default"() -> ()  [unwired: 3 in, 3 out]
            n65 = call <userlib>:"Fit VI window to Largest Dec__ogtk.vi"("error in (no error)"=w189, "border spacing (2 px)"=0) -> ("error out"=w188:errorcluster)  [unwired: 4 in, 1 out]
            n66 = call <vilib>:"Add State(s) to Queue__jki_lib_state_machine.vi"("State(s) in (\"\")"=w193) -> ("States Out"=w192:string)  [unwired: 14 in]
          }
          frame "UI: Update FP Controls" {
            # "Do not put any code in this frame.\n(It is a separator no-op. You can make a copy of this frame to create a new UI frame)"
            n67 = Unbundle By Name(w196) -> ("UI Cluster.Parameter"=w194:dbl, "UI Cluster.Parameter 2"=w195:string)
            n68 = local write "Parameter 2"(w195) -> ()
            n69 = local write "Parameter"(w194) -> ()
            n70 = call <vilib>:"Add State(s) to Queue__jki_lib_state_machine.vi"("State(s) in (\"\")"=w200) -> ("States Out"=w199:string)  [unwired: 14 in]
          }
          frame "UI: Update FP Indicators" {
            # "do this way to have nicer UI or only display what you want"
            n71 = Unbundle By Name(w201) -> ("getAll"=w203:T5)
            n72 = Unbundle By Name(w203) -> ("Levy 1"=→"Levy 1":dbl, "Logger SMO"=→"Logger SMO":dbl, "SMO Boolean"=→"SMO Boolean":bool, "SMO String"=→"SMO string":string)
            n73 = call <vilib>:"Add State(s) to Queue__jki_lib_state_machine.vi"("State(s) in (\"\")"=w210) -> ("States Out"=w209:string)  [unwired: 14 in]
          }
          frame "UI: Cursor Set" {
            # "Argument"
            # "Initialize the User Interface, here.\n(this is called automatically, by the Macro: Init)"
            n74 = disable-structure shown="Default" {
              disable-tunnel: w213 -> [w218 w221]
              disable-tunnel: [w218 w220] -> w212
              disable-tunnel: w211 -> [_ w219]
              frame condition #0 {
              }
              frame condition #1 (active) {
                n75 = case shown="\"Busy\"" w219 {
                  tunnel: w221 -> [w223 w225]
                  tunnel: [w222 w224] -> w220
                  frame "Idle", Default {
                    n76 = call <vilib>:"Unset Busy.vi"("error in (no error)"=w223) -> ("error out"=w222:errorcluster)  [unwired: 10 in]
                  }
                  frame "Busy" {
                    n77 = call <vilib>:"Set Busy.vi"("error in (no error)"=w225) -> ("error out"=w224:errorcluster)  [unwired: 9 in, 1 out]
                  }
                }
              }
            }
            n78 = call <vilib>:"Add State(s) to Queue__jki_lib_state_machine.vi"("State(s) in (\"\")"=w217) -> ("States Out"=w216:string)  [unwired: 14 in]
          }
          frame "UI: Front Panel State" {
            # "Argument"
            # "Set Front Panel Open or Closed\n(Usage: \"UI: Front Panel State >> Open|Close\")"
            n79 = Unbundle By Name(w229) -> ("Core.Current VI Reference"=w228:refnum<vi>)
            n80 = disable-structure shown="Default" {
              disable-tunnel: w231 -> [w237 w260]
              disable-tunnel: [w236 w260] -> w230
              disable-tunnel: w228 -> [w235 _]
              disable-tunnel: w227 -> [w234 _]
              frame condition #0 (active) {
                n81 = case shown="\"Close\"" w234 {
                  tunnel: w237 -> [w241 w254]
                  tunnel: [w243 w255] -> w236
                  tunnel: w235 -> [w242 w252]
                  frame "Open", Default {
                    n82 = property class="VI"(reference=w242, error in=w241) -> (reference out=w239:refnum<vi>, error out=w240:errorcluster, "FP.State"=w238:T2)
                    n83 = case shown="\"Closed\"" w238 {
                      tunnel: [w246 w249] -> w243
                      tunnel: w240 -> [w245 w249]
                      tunnel: w239 -> [w244 _]
                      frame "Closed" {
                        n84 = invoke class="VI" method="FP.Open"(reference=w244, error in=w245, "Activate"=TRUE, "State"=T2."Standard") -> (error out=w246:errorcluster)  [unwired: 1 in, 4 out]
                      }
                      frame Default {
                      }
                    }
                  }
                  frame "Close" {
                    n85 = property class="VI"(reference=w252, error in=w254) -> (reference out=w251:refnum<vi>, error out=w253:errorcluster, "FP.State"=w250:T2)
                    n86 = case shown="Default" w250 {
                      tunnel: [w256 w259] -> w255
                      tunnel: w253 -> [w256 w258]
                      tunnel: w251 -> [_ w257]
                      frame "Invalid", "Closed" {
                      }
                      frame Default {
                        n87 = invoke class="VI" method="FP.Close"(reference=w257, error in=w258) -> (error out=w259:errorcluster)  [unwired: 1 in, 2 out]
                      }
                    }
                  }
                }
              }
              frame condition #1 {
              }
            }
            n88 = call <vilib>:"Add State(s) to Queue__jki_lib_state_machine.vi"("State(s) in (\"\")"=w233) -> ("States Out"=w232:string)  [unwired: 14 in]
          }
          frame "---------- Macro ----------" {
            # "Do not put any code in this frame.\n(It is a separator no-op. You can make a copy of this frame to create a new Macro frame)"
            n89 = call <vilib>:"Add State(s) to Queue__jki_lib_state_machine.vi"("State(s) in (\"\")"=w265) -> ("States Out"=w264:string)  [unwired: 14 in]
          }
          frame "Macro: Initialize" {
            w268 = "UI: Initialize\nMacro: Read UI Config\nAction: Open\n//UI: Front Panel State >> Open"  # UI: Initialize Macro: Read UI Config Action: Open //UI: Front Panel State >> Open
            # "Initialization Macro\n(This is called once, when the VI starts)"
            n90 = call <vilib>:"Add State(s) to Queue__jki_lib_state_machine.vi"("State(s) in Front (\"\")"="Data: Initialize\nInitialize Core Data\nEvents: Register", "State(s) in (\"\")"="Process: Sync", "State(s) at Back (\"\")"=w268) -> ("States Out"=w267:string)  [unwired: 12 in]
            n91 = call <vilib>:"Add State(s) to Queue__jki_lib_state_machine.vi"("State(s) in Front (\"\")"=w267, "State(s) in (\"\")"=w274) -> ("States Out"=w273:string)  [unwired: 13 in]
          }
          frame "Macro: Post Error Handling" {
            # "Clear Last Error?"
            n92 = Unbundle By Name(w276) -> ("Core.Last Error.remaining states"=w278:string, "Core.Shutdown?"=w279:bool)
            n93 = Unbundle By Name(w276) -> ("Core.Last Error.error"=w282:errorcluster)
            n94 = case shown="False" FALSE {
              tunnel: w282 -> [w290 _]
              tunnel: [w290 _] -> w281
              frame False {
              }
              frame True {
              }
            }
            n95 = case shown="True" w279 {
              tunnel: w278 -> [w287 w289]
              tunnel: [w287 w288] -> w275
              frame False {
                # "These are the remaining states (at the moment the error occured). States can be altered according to business logic."
                # "NOT SHUTTING DOWN"
              }
              frame True {
                # "Developer can decide to alter the states but should be aware that during the shutdown process, there are certain states that must be run for the SMO to properly shut itself (and this process) down. As such, one can add states to perform additional clean-ups, but should append the remaining state to be executed."
                # "SHUTTING DOWN"
                n96 = call <vilib>:"Add State(s) to Queue__jki_lib_state_machine.vi"("State(s) in (\"\")"=w289) -> ("States Out"=w288:string)  [unwired: 14 in]
              }
            }
            n97 = Bundle By Name(cluster=w276, "Core.Last Error.error"=w281) -> (w277:T7)
            n98 = call <vilib>:"Add State(s) to Queue__jki_lib_state_machine.vi"("State(s) in Front (\"\")"=w275, "State(s) in (\"\")"=w286) -> ("States Out"=w285:string)  [unwired: 13 in]
          }
          frame "Macro: Read UI Config" {
            # "Do not put any code in this frame.\n(It is a separator no-op. You can make a copy of this frame to create a new Macro frame)"
            n99 = call <vilib>:"Add State(s) to Queue__jki_lib_state_machine.vi"("State(s) in Front (\"\")"="Configuration: Initialize\nConfiguration: Read UI Config File\nUI: Update FP Controls" ("State(s) in Front (\"\")"), "State(s) in (\"\")"=w296) -> ("States Out"=w295:string)  [unwired: 13 in]
          }
          frame "Macro: Write UI Config" {
            # "Do not put any code in this frame.\n(It is a separator no-op. You can make a copy of this frame to create a new Macro frame)"
            n100 = call <vilib>:"Add State(s) to Queue__jki_lib_state_machine.vi"("State(s) in Front (\"\")"="Data: Set UI Cluster\nConfiguration: Write UI Config File" ("State(s) in Front (\"\")"), "State(s) in (\"\")"=w302) -> ("States Out"=w301:string)  [unwired: 13 in]
          }
          frame "Macro: Exit" {
            # "Exit Macro\n(This is called once, when the VI exits)"
            n101 = Unbundle By Name(w304) -> ("Core.Close Panel on Exit?"=w314:bool)
            n102 = Select(t="UI: Front Panel State >> Close", s=w314, f="") -> (s? t:f=w311:string)
            n103 = call <vilib>:"Add State(s) to Queue__jki_lib_state_machine.vi"("State(s) in Front (\"\")"="Data: Cleanup\nEvents: Unregister\nProcess: Self Terminate", "State(s) in (\"\")"="Process: Sync", "State(s) at Back (\"\")"="Exit") -> ("States Out"=w306:string)  [unwired: 12 in]
            n104 = call <vilib>:"Add State(s) to Queue__jki_lib_state_machine.vi"("State(s) in Front (\"\")"="Action: Close\nMacro: Write UI Config", "State(s) in (\"\")"=w311, "State(s) at Back (\"\")"=w306) -> ("States Out"=w310:string)  [unwired: 12 in]
            n105 = call <vilib>:"Add State(s) to Queue__jki_lib_state_machine.vi"("State(s) in Front (\"\")"=w310, "State(s) in (\"\")"=w317) -> ("States Out"=w316:string)  [unwired: 13 in]
          }
          frame "---------- Process ----------" {
            # "Template Separator\n(You can make a copy of, or modify, this frame)"
            n106 = call <vilib>:"Add State(s) to Queue__jki_lib_state_machine.vi"("State(s) in (\"\")"=w322) -> ("States Out"=w321:string)  [unwired: 14 in]
          }
          frame "Process: Sync" {
            n107 = Unbundle By Name(w330) -> ("Instrument UI"=w326:refnum<class "Instrument UI.Framework-Template.lvclass">)
            n108 = call <vilib>:"WaitOnProcessSync.vi"("error in (no error)"=w325, "SMO"=w326) -> ("error out"=w324:errorcluster, "Don't run?"=w329:bool)  [unwired: 7 in, 1 out]
            n109 = Select(t="Data: Cleanup\nEvents: Unregister\nExit", s=w329, f="") -> (s? t:f=w323:string)
            n110 = call <vilib>:"Add State(s) to Queue__jki_lib_state_machine.vi"("State(s) in Front (\"\")"=w323, "State(s) in (\"\")"=w333) -> ("States Out"=w332:string)  [unwired: 13 in]
          }
          frame "Process: Self Terminate" {
            n111 = Unbundle By Name(w335) -> ("Instrument UI"=w334:refnum<class "Instrument UI.Framework-Template.lvclass">)
            n112 = call <vilib>:"SelfTerminate.vi"("error in (no error)"=w337, "SMO in"=w334) -> ("error out"=w336:errorcluster)  [unwired: 8 in, 1 out]
            n113 = call <vilib>:"Add State(s) to Queue__jki_lib_state_machine.vi"("State(s) in (\"\")"=w340) -> ("States Out"=w339:string)  [unwired: 14 in]
          }
          frame "---------- Events ----------" {
            # "Template Separator\n(You can make a copy of, or modify, this frame)"
            n114 = call <vilib>:"Add State(s) to Queue__jki_lib_state_machine.vi"("State(s) in (\"\")"=w345) -> ("States Out"=w344:string)  [unwired: 14 in]
          }
          frame "Events: Register" {
            # "Expand to add\nmore events"
            # "Base Class Protected Events"
            n115 = Unbundle By Name(w356) -> ("Instrument UI"=w347:refnum<class "Instrument UI.Framework-Template.lvclass">, "Instrument"=w346:refnum<class "Instrument.Framework-Template.lvclass">)
            n116 = call <vilib>:"GetProtectedEvents.vi"("SMO"=w347) -> ("error out"=w350:errorcluster, "SMO Protected Events"=w354:T9)  [unwired: 8 in, 1 out]
            n117 = call <userlib>:"Instrument.GetPublicEvents.vi"("Instrument"=w346) -> ("error out"=w348:errorcluster, "Instrument Public Events"=w349:T10)  [unwired: 8 in, 1 out]
            n118 = register-events(w354, w349) -> (reference out=w355:refnum<event-registration>, error out=w352:errorcluster)  [unwired: 2 in]
            n119 = Merge Errors(w348, w353, w352, w350) -> (w351:errorcluster)
            n120 = call <vilib>:"Add State(s) to Queue__jki_lib_state_machine.vi"("State(s) in (\"\")"=w358) -> ("States Out"=w357:string)  [unwired: 14 in]
          }
          frame "Events: Unregister" {
            n121 = Unregister For Events(event registration refnum=w361, error in=w360) -> (error out=w359:errorcluster)
            n122 = call <vilib>:"Add State(s) to Queue__jki_lib_state_machine.vi"("State(s) in (\"\")"=w364) -> ("States Out"=w363:string)  [unwired: 14 in]
          }
          frame "---------- Configuration ----------" {
            # "Do not put any code in this frame.\n(It is a separator no-op. You can make a copy of this frame to create a new UI frame)"
            n123 = call <vilib>:"Add State(s) to Queue__jki_lib_state_machine.vi"("State(s) in (\"\")"=w369) -> ("States Out"=w368:string)  [unwired: 14 in]
          }
          frame "Configuration: Initialize" {
            # "Do not put any code in this frame.\n(It is a separator no-op. You can make a copy of this frame to create a new UI frame)"
            n124 = Unbundle By Name(w377) -> ("Configuration"=w375:refnum<class "Configuration.lvclass">, "Instrument"=w376:refnum<class "Instrument.Framework-Template.lvclass">)
            n125 = call <vilib>:"GetName.vi"("error in (no error)"=w379, "SMO"=w376) -> ("error out"=w378:errorcluster, "Name"=w380:string)  [unwired: 6 in, 2 out]
            n126 = call <userlib>:"Default Path.vi"("error in (no error)"=w378, "Folder Name [Application Name]"=w380, "Configuration in"=w375) -> ("error out"=w371:errorcluster, "Configuration out"=w374:refnum<class "Configuration.lvclass">)  [unwired: 7 in]
            n127 = call <userlib>:"Write Section.vi"("error in (no error)"=w371, "Section"="UI", "Configuration in"=w374) -> ("error out"=w370:errorcluster, "Configuration out"=w373:refnum<class "Configuration.lvclass">)  [unwired: 7 in]
            n128 = Bundle By Name(cluster=w377, "Configuration"=w373) -> (w381:T7)
            n129 = call <vilib>:"Add State(s) to Queue__jki_lib_state_machine.vi"("State(s) in (\"\")"=w384) -> ("States Out"=w383:string)  [unwired: 14 in]
          }
          frame "Configuration: Write UI Config File" {
            # "Do not put any code in this frame.\n(It is a separator no-op. You can make a copy of this frame to create a new Data frame)"
            n130 = Unbundle By Name(w389) -> ("Configuration"=w386:refnum<class "Configuration.lvclass">, "UI Cluster"=w388:T6)
            n131 = call <userlib>:"Write Configuration.vi"("error in (no error)"=w385, "Variant"=w388, "Configuration in"=w386) -> ("error out"=w387:errorcluster)  [unwired: 7 in, 1 out]
            n132 = call <vilib>:"Add State(s) to Queue__jki_lib_state_machine.vi"("State(s) in (\"\")"=w392) -> ("States Out"=w391:string)  [unwired: 14 in]
          }
          frame "Configuration: Read UI Config File" {
            # "Do not put any code in this frame.\n(It is a separator no-op. You can make a copy of this frame to create a new UI frame)"
            n133 = Unbundle By Name(w395) -> ("UI Cluster"=w398:T6, "Configuration"=w401:refnum<class "Configuration.lvclass">)
            n134 = call <userlib>:"Read Configuration.vi"("INI Fomatted Cluster Type"=w398, "error in (no error)"=w397, "Configuration in"=w401) -> ("error out"=w400:errorcluster, "Configuration"=w399:variant)  [unwired: 6 in, 1 out]
            n135 = Variant To Data(error in=w400, type=w398, Variant=w399) -> (data=w394:T6, error out=w396:errorcluster)
            n136 = Bundle By Name(cluster=w395, "UI Cluster"=w394) -> (w393:T7)
            n137 = call <vilib>:"Add State(s) to Queue__jki_lib_state_machine.vi"("State(s) in (\"\")"=w404) -> ("States Out"=w403:string)  [unwired: 14 in]
          }
          frame "---------- Action ----------" {
            n138 = Unbundle By Name(w407) -> ("Instrument UI"=w405:refnum<class "Instrument UI.Framework-Template.lvclass">)
            n139 = Bundle By Name(cluster=w407, "Instrument UI"=w405) -> (w406:T7)
            n140 = call <vilib>:"Add State(s) to Queue__jki_lib_state_machine.vi"("State(s) in (\"\")"=w411) -> ("States Out"=w410:string)  [unwired: 14 in]
          }
          frame "Action: Notify UI Closed" {
            # "Notify that the UI has been closed"
            n141 = Unbundle By Name(w412) -> ("Instrument UI"=w415:refnum<class "Instrument UI.Framework-Template.lvclass">)
            n142 = call <vilib>:"Hide.vi"("error in (no error)"=w414, "SMO.UI"=w415) -> ("error out"=w413:errorcluster)  [unwired: 8 in, 1 out]
            n143 = call <vilib>:"Add State(s) to Queue__jki_lib_state_machine.vi"("State(s) in (\"\")"=w418) -> ("States Out"=w417:string)  [unwired: 14 in]
          }
          frame "Action: getAll" {
            n144 = Unbundle By Name(w422) -> ("getAll"=w420:T5, "Instrument"=w425:refnum<class "Instrument.Framework-Template.lvclass">)
            n145 = call "GET ALL.vim"("type"=w420, "error in (no error)"=w423, "Instrument in"=w425) -> ("error out"=w427:errorcluster, "getAll"=w419:T5, "Instrument out"=w421:refnum<class "Instrument.Framework-Template.lvclass">)  [unwired: 6 in]
            n146 = Bundle By Name(cluster=w422, "Instrument"=w421, "getAll"=w419) -> (w424:T7)
            n147 = call <vilib>:"Add State(s) to Queue__jki_lib_state_machine.vi"("State(s) in Front (\"\")"="" ("State(s) in Front (\"\")"), "State(s) in (\"\")"=w430) -> ("States Out"=w429:string)  [unwired: 13 in]
          }
          frame "Action: Open" {
            n148 = Unbundle By Name(w437) -> ("Instrument"=w435:refnum<class "Instrument.Framework-Template.lvclass">)
            n149 = call <userlib>:"Write Client Type.vi"("error in (no error)"=w432, "Client Type"=Client_Type--Enum."Local", "Instrument in"=w435) -> ("error out"=w433:errorcluster, "Instrument out"=w434:refnum<class "Instrument.Framework-Template.lvclass">)  [unwired: 7 in]
            n150 = call-dynamic "Open.vi"("error in (no error)"=w433, "Instrument.Template in"=w434) -> ("error out"=w440:errorcluster, "Instrument.Template out"=w436:refnum<class "Instrument.Framework-Template.lvclass">)  [unwired: 8 in]
            n151 = Bundle By Name(cluster=w437, "Instrument"=w436) -> (w438:T7)
            n152 = call <vilib>:"Add State(s) to Queue__jki_lib_state_machine.vi"("State(s) in Front (\"\")"="" ("State(s) in Front (\"\")"), "State(s) in (\"\")"=w443) -> ("States Out"=w442:string)  [unwired: 13 in]
          }
          frame "Action: Close" {
            n153 = Unbundle By Name(w445) -> ("Instrument"=w448:refnum<class "Instrument.Framework-Template.lvclass">)
            n154 = call-dynamic "Close.vi"("error in (no error)"=w446, "Instrument.Template in"=w448) -> ("error out"=w450:errorcluster, "Instrument.Template out"=w444:refnum<class "Instrument.Framework-Template.lvclass">)  [unwired: 8 in]
            n155 = Bundle By Name(cluster=w445, "Instrument"=w444) -> (w447:T7)
            n156 = call <vilib>:"Add State(s) to Queue__jki_lib_state_machine.vi"("State(s) in Front (\"\")"="" ("State(s) in Front (\"\")"), "State(s) in (\"\")"=w453) -> ("States Out"=w452:string)  [unwired: 13 in]
          }
          frame "Action: setConfiguration" {
            n157 = Unbundle By Name(w456) -> ("Instrument"=w459:refnum<class "Instrument.Framework-Template.lvclass">, "Config Cluster"=w454:T4)
            n158 = call "SET CONFIG.vim"("error in (no error)"=w457, "Configuration"=w454, "Instrument in"=w459) -> ("error out"=w461:errorcluster, "Instrument out"=w455:refnum<class "Instrument.Framework-Template.lvclass">)  [unwired: 7 in]
            n159 = Bundle By Name(cluster=w456, "Instrument"=w455) -> (w458:T7)
            n160 = call <vilib>:"Add State(s) to Queue__jki_lib_state_machine.vi"("State(s) in Front (\"\")"="" ("State(s) in Front (\"\")"), "State(s) in (\"\")"=w464) -> ("States Out"=w463:string)  [unwired: 13 in]
          }
        }
      }
    }
    frame Error {
    }
  }
  n161 = call-parent "Process.vi"("error in"=w5, "Instrument UI in"=w4) -> ("error out"=w2:errorcluster, "Instrument UI out"=→"Example Instrument UI out":refnum<class "Instrument UI.Framework-Template.lvclass">)  [unwired: 8 in]
  n162 = Merge Errors(w2, w1) -> (→"error out":errorcluster)
